vi "Multiply Output Gain.vi"(8 "error in (no error)":errorcluster, 10 "WFM in":waveform(dbl)[](array[waveform]), 11 "Instrument.DAQ":refnum<class "Instrument.DAQ.lvclass">) -> (0 "error out":errorcluster, 2 "WFM out":waveform(dbl)[](array[waveform]), 3 "Instrument.DAQ out":refnum<class "Instrument.DAQ.lvclass">)   [LabVIEW 2019, in "Instrument.Lockin.lvlib" / "Instrument.DAQ.lvclass"]
uses:
  Instrument.DAQ.lvclass
  Instrument.DAQ.lvclass/Instrument.DAQ.ctl
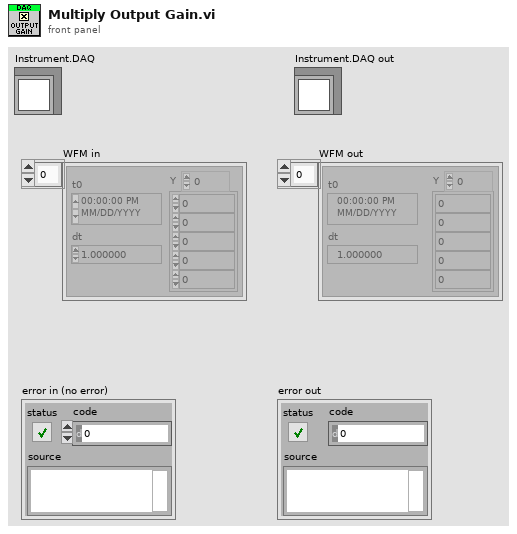
[diagram p1: front panel]
types:
  T1 = typedef "Instrument.Lockin.lvlib/Instrument.DAQ.lvclass/Channel.Gain--Cluster--Array.ctl" = T2[]
  T2 = typedef "Instrument.Lockin.lvlib/Instrument.DAQ.lvclass/Channel.Gain--Cluster.ctl" = cluster{"Channel":string, "Gain":dbl}
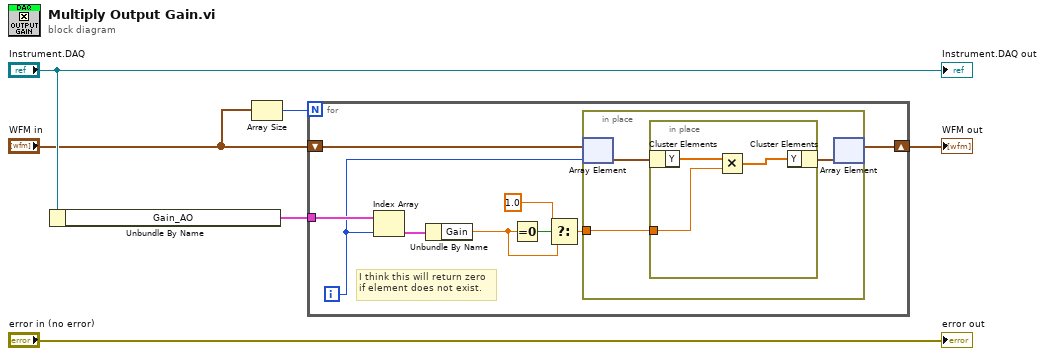
[diagram p0: block diagram]
diagram:
  n1 = Unbundle By Name("Instrument.DAQ") -> ("Gain_AO"=w1:T1)
  n2 = Array Size(array="WFM in") -> (size(s)=w2:i32)
  n3 = for {
    N: w2 -> [_]
    tunnel: w1 -> [w11]
    shift-right: [w15] -> w6
    shift-left: "WFM in" -> [w14]
    i -> [w9]
    # "I think this will return zero\nif element does not exist."
    n4 = Index Array(array=w11, index=w9) -> (element=w8:T2)
    n5 = Unbundle By Name(w8) -> ("Gain"=w7:dbl)
    n6 = Equal To 0?(x=w7) -> (x = 0?=w13:bool)
    n7 = Select(t=1.0, s=w13, f=w7) -> (s? t:f=w10:dbl)
    n8 = in-place {
      in-place-border: w10 -> [w18]
      n9 = in-place-array #1(w14, w9) -> (w17:waveform(dbl))
      n10 = in-place {
        in-place-border: w18 -> [w21]
        n11 = in-place-cluster #2(w17) -> ("Y"=w20:dbl[])
        n12 = Multiply(x=w20, y=w21) -> (x*y=w19:dbl[])
        n13 = in-place-cluster #2("Y"=w19) -> (w16:waveform(dbl))
      }
      n14 = in-place-array #1(w16) -> (w15:waveform(dbl)[])  [unwired: 1 out]
    }
  }
  "WFM out" <- w6
  "error out" <- "error in (no error)"
  "Instrument.DAQ out" <- "Instrument.DAQ"
